vi "NovRAM Write.vi"(8 "error in (no error)":errorcluster, 9 "WORD TO WRITE":u16 step=1 format="%.0x", 10 "NOVRAM ADDRESS":u8=1 min=1 max=64 step=1, 11 "VISA resource name":refnum<visa-resource-name>) -> (0 "error out":errorcluster, 3 "VISA resource name out":refnum<visa-resource-name>)   [LabVIEW 2009, in "Digikrom DK24x.lvlib"]
doc: "Writes a word (0 to 65535) to a Novram address (1 to 64) indicated by address byte.\n\nWARNING !!!\nImproper use of this command may corrupt the configuration and calibration information of the monochromator. See ‘Restore Disk’ supplied to restore values."
uses:
  Digikrom DK24x.lvlib
  Private/Command.ctl
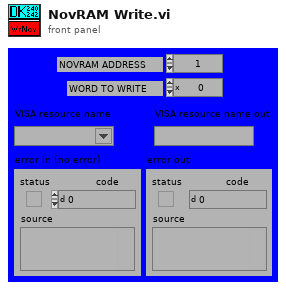
[diagram p1: front panel]
types:
  T1 = typedef "Digikrom DK24x.lvlib/Command.ctl" = u8
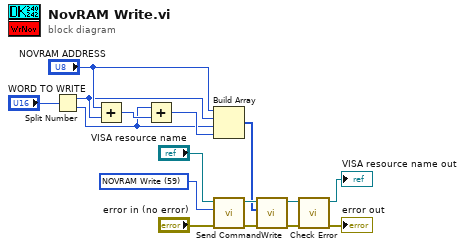
[diagram p0: block diagram]
diagram:
  w1 = T1 59 items=["Cancel"=24, "Clear"=25, "CSR"=28, "Echo"=27, "Filter"=15, "Gcal"=18, "Goto"=16, "Grtid?"=19, "Grtsel"=26, "NOVRAM Read"=56, "NOVRAM Write"=59, "Reset"=255, "Scan"=12, "Scan Up"=9, "Scan Down"=3, "Serial?"=33, "Slew Up"=8, "Slew Down"=2, "Slit Reset"=43, "Slit?"=30, "Sltadj"=14, "Speed"=13, "Sspeed?"=21, "Step Down"=1, "Step Up"=7, "S1adj"=31, "S2adj"=32, "S3adj"=34, "S1cal"=22, "S2cal"=23, "S3cal"=35, "Test"=17, "Type"=57, "Wave?"=29, "Zero"=52] ("Command")
  n1 = Split Number(x="WORD TO WRITE") -> (hi(x)=w13:u8, lo(x)=w11:u8)
  n2 = Add(x="NOVRAM ADDRESS", y=w13) -> (x+y=w12:u8)
  n3 = Add(x=w11, y=w12) -> (x+y=w14:u8)
  n4 = Build Array("NOVRAM ADDRESS", w13, w11, w14) -> (w2:u8[])
  n5 = call "Send Command.vi"("error in (no error)"="error in (no error)", "Command"=w1, "VISA resource name"="VISA resource name") -> ("error out"=w5:errorcluster, "VISA resource name out"=w6:refnum<visa-resource-name>)  [unwired: 7 out]
  n6 = call "Write.vi"("error in (no error)"=w5, "Byte Array"=w2, "VISA resource name"=w6) -> ("error out"=w10:errorcluster, "VISA resource name out"=w9:refnum<visa-resource-name>)  [unwired: 7 out]
  n7 = call "Check Error.vi"("error in"=w10, "VISA resource name in"=w9) -> ("error out"=→"error out":errorcluster, "VISA resource name out"=→"VISA resource name out":refnum<visa-resource-name>)  [unwired: 1 in, 7 out]
